vi "digitally_ros_without_joystick_debugging.vi"() -> ()   [LabVIEW 2019]
uses:
  <vilib>/addons/eal4LabVIEW/ApiLib/Connection control/ealApiConnect_string.vi
  <vilib>/addons/eal4LabVIEW/eal4LabVIEW.lvlib
panel:
  out "PID return":dbl[](array[numeric])
  out "output cluster 3":cluster{"upper limit":dbl, dbl, dbl, dbl}
  out "output cluster 2":cluster{"upper limit":dbl, dbl, dbl, dbl}
  out "output cluster":cluster{"upper limit":dbl, dbl, dbl, dbl}
  out "I value":i32
  out "error out":errorcluster
  out "Is the PID fnished?":bool[](array[boolean])
  out "In Range? (1)":bool
  out "In Range? (2)":bool
  out "In Range? (3)":bool
  in  "condition 6":i32(ring) items=["AXIS_CONDITION_ACTIVE"=0, "AXIS_CONDITION_PARKING"=1, "AXIS_CONDITION_DEACTIVATED"=2, "AXIS_CONDITION_ACTIVE_DECOUPLED"=4, "AXIS_CONDITION_PARKING_DECOUPLED"=5, "AXIS_CONDITION_DEACTIVATED_DECOUPLED"=6, "AXIS_CONDITION_ACTIVE_PARAMETERIZATION"=8, "AXIS_CONDITION_PARKING_PARAMETERIZATION"=9, "AXIS_CONDITION_DEACTIVATED_PARAMETERIZATION"=10, "AXIS_CONDITION_ACTIVE_DECOUPLED_PARAMETERIZATION"=12, "AXIS_CONDITION_PARKING_DECOUPLED_PARAMETERIZATION"=13, "AXIS_CONDITION_DEACTIVATED_DECOUPLED_PARAMETERIZATION"=14]
  in  "slave index 6":i32
  in  "condition 5":i32(ring) items=["AXIS_CONDITION_ACTIVE"=0, "AXIS_CONDITION_PARKING"=1, "AXIS_CONDITION_DEACTIVATED"=2, "AXIS_CONDITION_ACTIVE_DECOUPLED"=4, "AXIS_CONDITION_PARKING_DECOUPLED"=5, "AXIS_CONDITION_DEACTIVATED_DECOUPLED"=6, "AXIS_CONDITION_ACTIVE_PARAMETERIZATION"=8, "AXIS_CONDITION_PARKING_PARAMETERIZATION"=9, "AXIS_CONDITION_DEACTIVATED_PARAMETERIZATION"=10, "AXIS_CONDITION_ACTIVE_DECOUPLED_PARAMETERIZATION"=12, "AXIS_CONDITION_PARKING_DECOUPLED_PARAMETERIZATION"=13, "AXIS_CONDITION_DEACTIVATED_DECOUPLED_PARAMETERIZATION"=14]
  in  "slave index 5":i32
  in  "condition 4":i32(ring) items=["AXIS_CONDITION_ACTIVE"=0, "AXIS_CONDITION_PARKING"=1, "AXIS_CONDITION_DEACTIVATED"=2, "AXIS_CONDITION_ACTIVE_DECOUPLED"=4, "AXIS_CONDITION_PARKING_DECOUPLED"=5, "AXIS_CONDITION_DEACTIVATED_DECOUPLED"=6, "AXIS_CONDITION_ACTIVE_PARAMETERIZATION"=8, "AXIS_CONDITION_PARKING_PARAMETERIZATION"=9, "AXIS_CONDITION_DEACTIVATED_PARAMETERIZATION"=10, "AXIS_CONDITION_ACTIVE_DECOUPLED_PARAMETERIZATION"=12, "AXIS_CONDITION_PARKING_DECOUPLED_PARAMETERIZATION"=13, "AXIS_CONDITION_DEACTIVATED_DECOUPLED_PARAMETERIZATION"=14]
  in  "slave index 4":i32
  out "RPM 1 ROS":dbl
  out "RPM 2 ROS":dbl
  out "RPM 3 ROS":dbl
  in  "stop":bool
  out "Return value":dbl[](array[numeric])
  out "Iteration counter":i32
  # "ROS Control"
  # "Joystick Control"
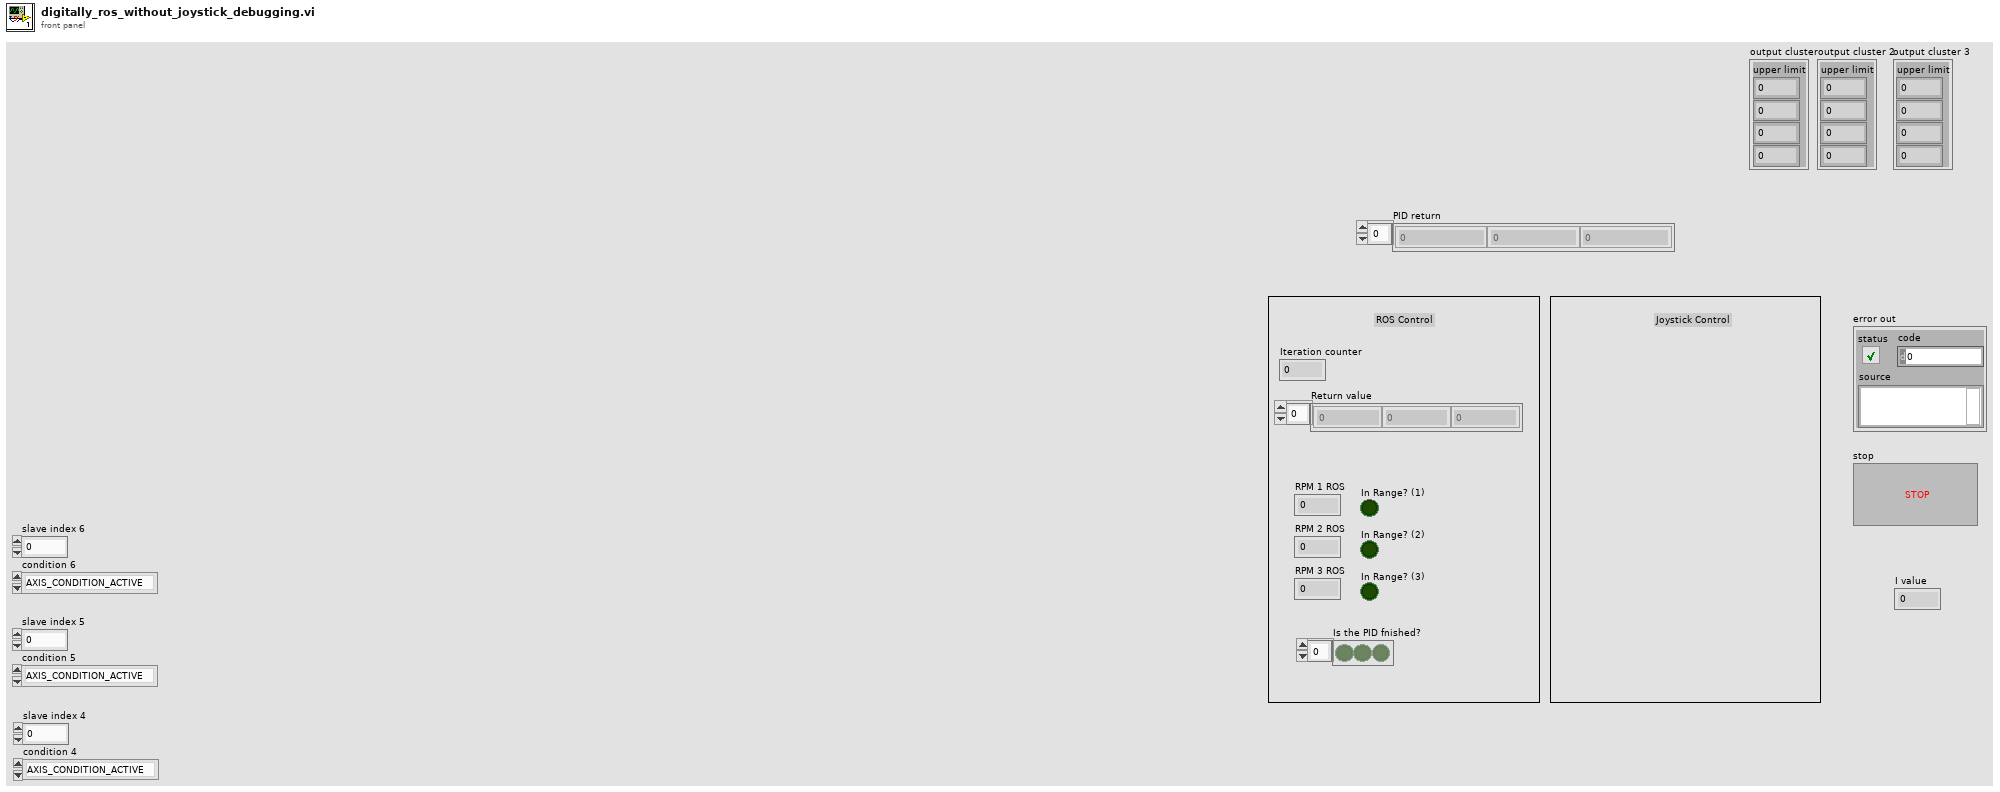
[diagram p1: front panel]
types:
  T1 = cluster{"Velocity":dbl, "Acceleration":dbl, "Deceleration":dbl, "Jerk":dbl}
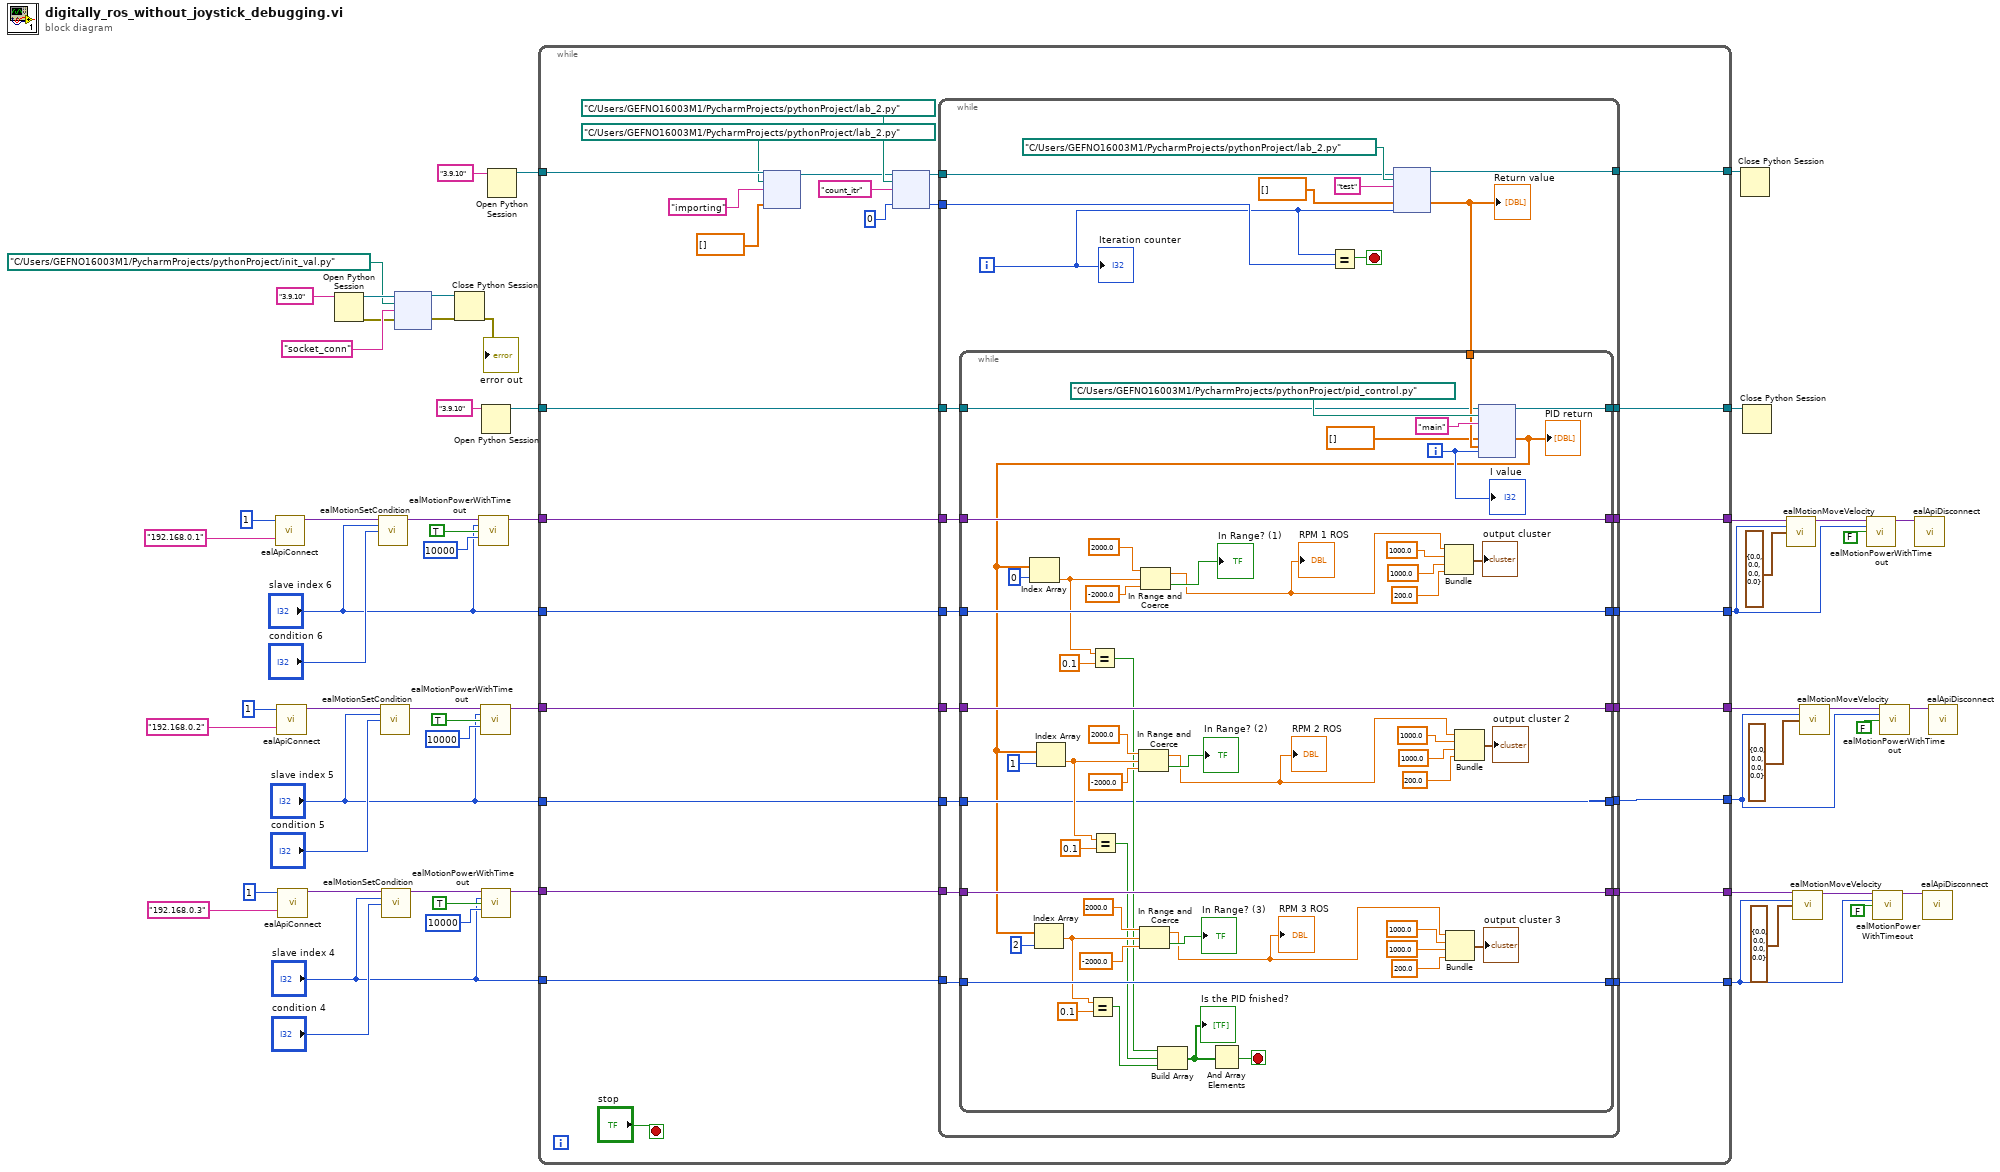
[diagram p0: block diagram]
diagram:
  n1 = call-poly <vilib>:"ealApiConnect.vi"("maximum no of axes"=1, "ip address"="192.168.0.1") -> ("connection out"=w31:variant)  [unwired: 12 in, 1 out]
  n2 = call-poly <vilib>:"ealApiConnect.vi"("maximum no of axes"=1, "ip address"="192.168.0.2") -> ("connection out"=w38:variant)  [unwired: 12 in, 1 out]
  n3 = call-poly <vilib>:"ealApiConnect.vi"("maximum no of axes"=1, "ip address"="192.168.0.3") -> ("connection out"=w45:variant)  [unwired: 12 in, 1 out]
  n4 = Open Python Session(python version="3.9.10" ("Python version")) -> (session out=w7:refnum<k35>, error out=w3:errorcluster)  [unwired: 2 in]
  n5 = call <vilib>:"ealMotionSetCondition.vi"("connection in"=w31, "slave index"="slave index 6", "condition"="condition 6") -> ("connection out"=w30:variant)  [unwired: 11 in, 1 out]
  n6 = call <vilib>:"ealMotionSetCondition.vi"("connection in"=w38, "slave index"="slave index 5", "condition"="condition 5") -> ("connection out"=w37:variant)  [unwired: 11 in, 1 out]
  n7 = call <vilib>:"ealMotionSetCondition.vi"("connection in"=w45, "slave index"="slave index 4", "condition"="condition 4") -> ("connection out"=w44:variant)  [unwired: 11 in, 1 out]
  n8 = node(w7, path "C:/Users/GEFNO16003M1/PycharmProjects/pythonProject/init_val.py" ("module path"), "socket_conn" ("function name"), w3) -> (w6:refnum<k35>, w2:errorcluster)  [unwired: 2 in, 2 out]
  n9 = Close Python Session(session in=w6, error in=w2) -> (11:→"error out":errorcluster)
  n10 = call <vilib>:"ealMotionPowerWithTimeout.vi"("connection in"=w30, "slave index"="slave index 6", "value"=TRUE, "timeout"=10000) -> ("connection out"=w26:variant)  [unwired: 10 in, 1 out]
  n11 = call <vilib>:"ealMotionPowerWithTimeout.vi"("connection in"=w37, "slave index"="slave index 5", "value"=TRUE, "timeout"=10000) -> ("connection out"=w25:variant)  [unwired: 10 in, 1 out]
  n12 = Open Python Session(python version="3.9.10" ("Python version")) -> (session out=w12:refnum<k35>)  [unwired: 2 in, 1 out]
  n13 = call <vilib>:"ealMotionPowerWithTimeout.vi"("connection in"=w44, "slave index"="slave index 4", "value"=TRUE, "timeout"=10000) -> ("connection out"=w24:variant)  [unwired: 10 in, 1 out]
  n14 = Open Python Session(python version="3.9.10" ("Python version")) -> (session out=w15:refnum<k35>)  [unwired: 2 in, 1 out]
  n15 = while {
    tunnel: w26 -> [w84]
    tunnel: w25 -> [w83]
    tunnel: w24 -> [w82]
    tunnel: [w69] -> w23
    tunnel: [w81] -> w22
    tunnel: "slave index 6" -> [w80]
    tunnel: "slave index 5" -> [w79]
    tunnel: [w78] -> w19
    tunnel: [w72] -> w18
    tunnel: "slave index 4" -> [w77]
    tunnel: w15 -> [w76]
    tunnel: [w75] -> w14
    tunnel: w12 -> [w74]
    tunnel: [w70] -> w11
    tunnel: [w73] -> w10
    tunnel: [w71] -> w9
    stop <- "stop" stop-if-true
    n16 = node(w76, path "C:/Users/GEFNO16003M1/PycharmProjects/pythonProject/lab_2.py" ("module path"), "importing" ("function name"), dbl[] []) -> (w63:refnum<k35>)  [unwired: 2 in, 3 out]
    n17 = node(w63, path "C:/Users/GEFNO16003M1/PycharmProjects/pythonProject/lab_2.py" ("module path"), "count_itr" ("function name"), 0) -> (w62:refnum<k35>, w60:i32)  [unwired: 1 in, 3 out]
    n18 = while {
      tunnel: [w102] -> w75
      tunnel: w62 -> [w105]
      tunnel: w60 -> [w103]
      tunnel: w84 -> [w100]
      tunnel: w83 -> [w89]
      tunnel: w82 -> [w99]
      tunnel: [w91] -> w69
      tunnel: [w92] -> w81
      tunnel: w80 -> [w90]
      tunnel: w79 -> [w88]
      tunnel: [w93] -> w78
      tunnel: w77 -> [w95]
      tunnel: w74 -> [w87]
      tunnel: [w97] -> w70
      tunnel: [w96] -> w73
      tunnel: [w94] -> w72
      tunnel: [w86] -> w71
      i -> [w98]
      stop <- w106 stop-if-true
      n19 = Equal?(x=w98, y=w103) -> (x = y?=w106:bool)
      n20 = node(w105, path "C:/Users/GEFNO16003M1/PycharmProjects/pythonProject/lab_2.py" ("module path"), "test" ("function name"), dbl[] [], w98) -> (w102:refnum<k35>, w101:dbl[])  [unwired: 2 in, 3 out]
      "Return value" <- w101
      n21 = while {
        tunnel: w101 -> [w158]
        tunnel: w100 -> [w133]
        tunnel: w99 -> [w135]
        tunnel: [w135] -> w97
        tunnel: [w134] -> w96
        tunnel: w95 -> [w134]
        tunnel: [w131] -> w94
        tunnel: [w113] -> w93
        tunnel: [w132] -> w92
        tunnel: [w133] -> w91
        tunnel: w90 -> [w132]
        tunnel: w89 -> [w131]
        tunnel: w88 -> [w113]
        tunnel: w87 -> [w130]
        tunnel: [w129] -> w86
        i -> [w114]
        stop <- w128 stop-if-true
        n22 = node(w130, path "C:/Users/GEFNO16003M1/PycharmProjects/pythonProject/pid_control.py" ("module path"), "main" ("function name"), dbl[] [], w158, w114) -> (w129:refnum<k35>, w109:dbl[])  [unwired: 3 in, 3 out]
        "PID return" <- w109
        n23 = Index Array(array=w109, index=0) -> (element=w124:dbl)
        n24 = Index Array(array=w109, index=2) -> (element=w122:dbl)
        n25 = Index Array(array=w109, index=1) -> (element=w123:dbl)
        n26 = Equal?(x=w122, y=0.1) -> (x = y?=w119:bool)
        n27 = Equal?(x=w124, y=0.1) -> (x = y?=w121:bool)
        n28 = Equal?(x=w123, y=0.1) -> (x = y?=w120:bool)
        n29 = In Range and Coerce(upper limit=2000.0, x=w123, lower limit=-2000.0) -> (coerced(x)=w116:dbl, In Range?=→"In Range? (2)":bool)
        "RPM 2 ROS" <- w116
        n30 = In Range and Coerce(upper limit=2000.0, x=w122, lower limit=-2000.0) -> (coerced(x)=w115:dbl, In Range?=→"In Range? (3)":bool)
        "RPM 3 ROS" <- w115
        n31 = In Range and Coerce(upper limit=2000.0, x=w124, lower limit=-2000.0) -> (coerced(x)=w117:dbl, In Range?=→"In Range? (1)":bool)
        "RPM 1 ROS" <- w117
        n32 = Build Array(w121, w120, w119) -> (w118:bool[])
        "Is the PID fnished?" <- w118
        n33 = And Array Elements(Boolean array=w118) -> (logical AND=w128:bool)
        n34 = Bundle("upper limit"=w117, 1000.0, 1000.0, 200.0) -> (→"output cluster":cluster{"upper limit":dbl, dbl, dbl, dbl})  [unwired: 1 in]
        n35 = Bundle("upper limit"=w115, 1000.0, 1000.0, 200.0) -> (→"output cluster 3":cluster{"upper limit":dbl, dbl, dbl, dbl})  [unwired: 1 in]
        n36 = Bundle("upper limit"=w116, 1000.0, 1000.0, 200.0) -> (→"output cluster 2":cluster{"upper limit":dbl, dbl, dbl, dbl})  [unwired: 1 in]
        "I value" <- w114
      }
      "Iteration counter" <- w98
    }
  }
  n37 = Close Python Session(session in=w14) -> ()  [unwired: 1 in, 1 out]
  n38 = Close Python Session(session in=w9) -> ()  [unwired: 1 in, 1 out]
  n39 = call <vilib>:"ealMotionMoveVelocity.vi"("connection in"=w23, "slave index"=w22, "parameters set"=T1 {"Velocity"=0.0, "Acceleration"=0.0, "Deceleration"=0.0, "Jerk"=0.0}) -> ("connection out"=w50:variant)  [unwired: 11 in, 1 out]
  n40 = call <vilib>:"ealMotionMoveVelocity.vi"("connection in"=w11, "slave index"=w10, "parameters set"=T1 {"Velocity"=0.0, "Acceleration"=0.0, "Deceleration"=0.0, "Jerk"=0.0}) -> ("connection out"=w58:variant)  [unwired: 11 in, 1 out]
  n41 = call <vilib>:"ealMotionMoveVelocity.vi"("connection in"=w18, "slave index"=w19, "parameters set"=T1 {"Velocity"=0.0, "Acceleration"=0.0, "Deceleration"=0.0, "Jerk"=0.0}) -> ("connection out"=w54:variant)  [unwired: 11 in, 1 out]
  n42 = call <vilib>:"ealMotionPowerWithTimeout.vi"("connection in"=w50, "slave index"=w22, "value"=FALSE) -> ("connection out"=w51:variant)  [unwired: 11 in, 1 out]
  n43 = call <vilib>:"ealMotionPowerWithTimeout.vi"("connection in"=w58, "slave index"=w10, "value"=FALSE) -> ("connection out"=w59:variant)  [unwired: 11 in, 1 out]
  n44 = call <vilib>:"ealMotionPowerWithTimeout.vi"("connection in"=w54, "slave index"=w19, "value"=FALSE) -> ("connection out"=w55:variant)  [unwired: 11 in, 1 out]
  n45 = call <vilib>:"ealApiDisconnect.vi"("connection in"=w51) -> ()  [unwired: 14 in, 1 out]
  n46 = call <vilib>:"ealApiDisconnect.vi"("connection in"=w59) -> ()  [unwired: 14 in, 1 out]
  n47 = call <vilib>:"ealApiDisconnect.vi"("connection in"=w55) -> ()  [unwired: 14 in, 1 out]
